vi "getStyleName.vi"(8 "error in (no error)":errorcluster, 11 "Font in":refnum<class "Heading 3.lvclass">) -> (0 "error out":errorcluster, 2 "Style Name":string, 3 "Font out":refnum<class "Heading 3.lvclass">)   [LabVIEW 2020, in "Styles.lvlib" / "Heading 3.lvclass"]
uses:
  Heading 3.lvclass
  Heading 3.lvclass/Heading 3.ctl
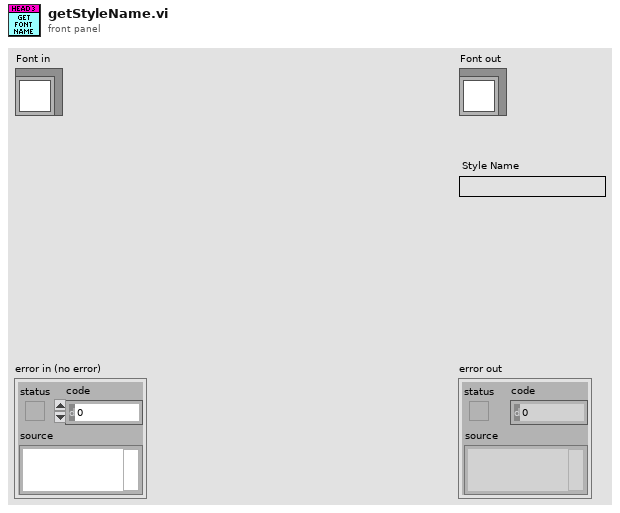
[diagram p1: front panel]
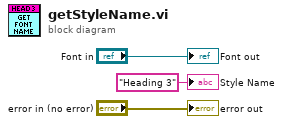
[diagram p0: block diagram]
diagram:
  "error out" <- "error in (no error)"
  "Font out" <- "Font in"
  "Style Name" <- "Heading 3" ("Style Name")
